vi "xy from XY.vi"(8 "error in (no error)":errorcluster, 11 "Data2D in":refnum<class "Data2D.lvclass">) -> (0 "error out":errorcluster, 1 "y":dbl, 2 "x":dbl, 3 "Data2D out":refnum<class "Data2D.lvclass">)   [LabVIEW 2014, in "Data2D.lvclass"]
uses:
  Data2D.lvclass
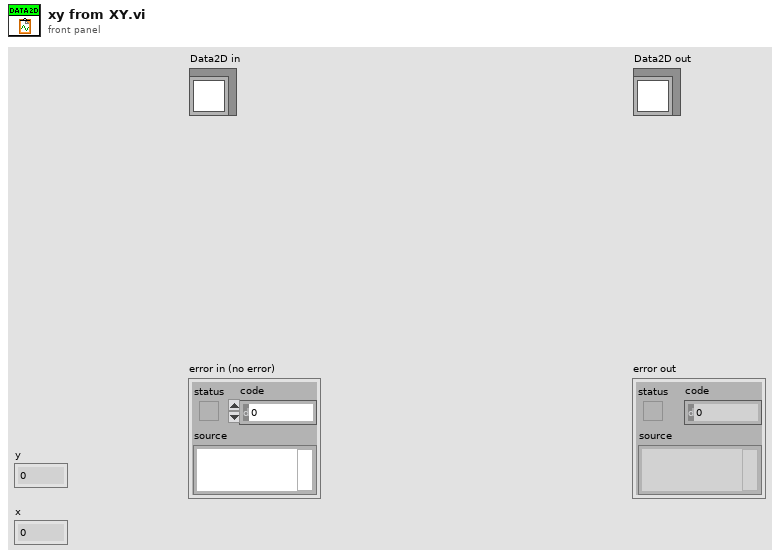
[diagram p1: front panel]
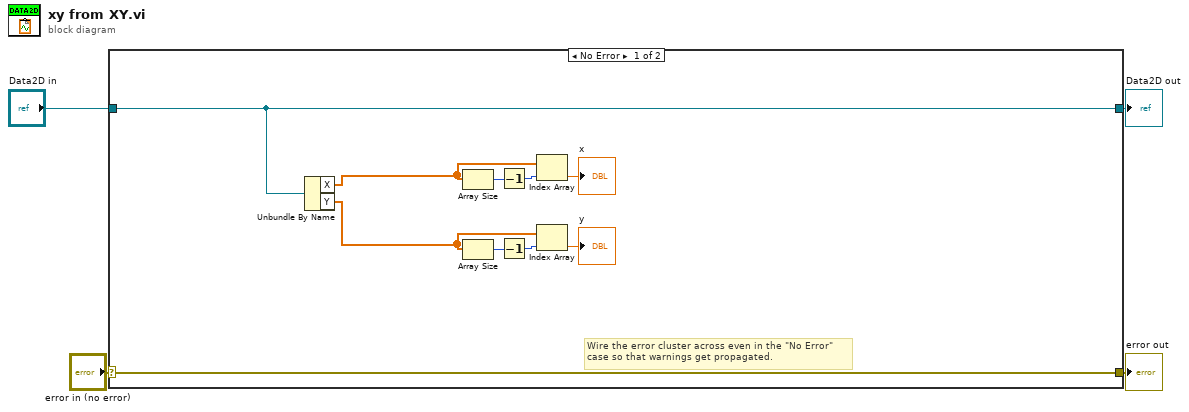
[diagram p0: block diagram]
diagram:
  n1 = case shown="No Error" "error in (no error)" {
    selector: "error in (no error)" -> [w14 w16]
    tunnel: [w14 w16] -> w3
    tunnel: [w7 w15] -> w1
    tunnel: "Data2D in" -> [w7 w15]
    frame No Error {
      # "Wire the error cluster across even in the \"No Error\"\ncase so that warnings get propagated."
      n2 = Unbundle By Name(w7) -> ("X"=w6:dbl[], "Y"=w5:dbl[])
      n3 = Array Size(array=w6) -> (size(s)=w11:i32)
      n4 = Array Size(array=w5) -> (size(s)=w8:i32)
      n5 = Decrement(x=w11) -> (x-1=w12:i32)
      n6 = Decrement(x=w8) -> (x-1=w9:i32)
      n7 = Index Array(array=w6, index=w12) -> (element=→"x":dbl)
      n8 = Index Array(array=w5, index=w9) -> (element=→"y":dbl)
    }
    frame Error {
    }
  }
  "error out" <- w3
  "Data2D out" <- w1
